vi "Write Mutation Type.vi"(8 "error in (no error)":errorcluster, 10 "Mutation Type":T1, 11 "GA in":refnum<class "GA.lvclass">) -> (0 "error out":errorcluster, 3 "GA out":refnum<class "GA.lvclass">)   [LabVIEW 2013, in "GA.lvclass"]
uses:
  GA.lvclass
  Controls/Mutation Type.ctl
  GA.lvclass/GA.ctl
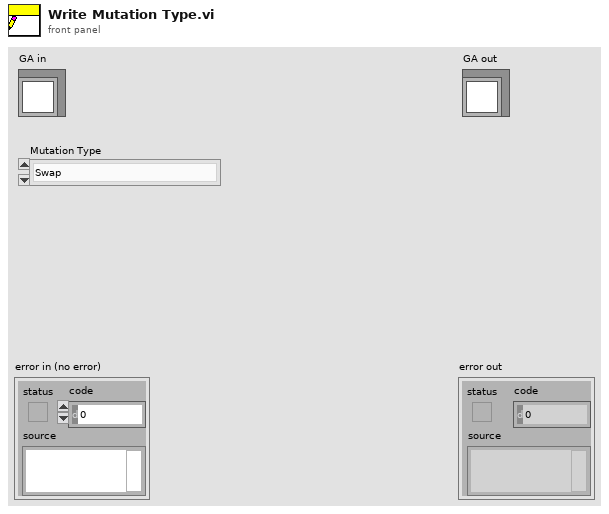
[diagram p1: front panel]
types:
  T1 = typedef "GA.lvclass/Mutation Type.ctl" = enum16{"Swap", "Insert", "Shift", "Shuflle", "Inversion", "ND Mutation"}
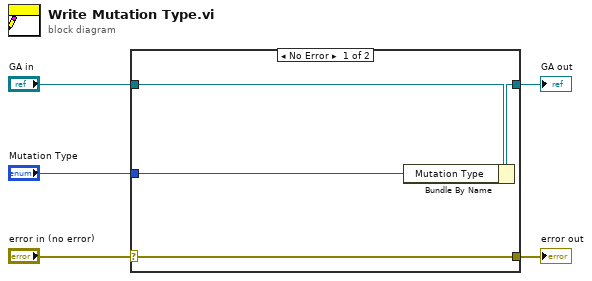
[diagram p0: block diagram]
diagram:
  n1 = case shown="No Error" "error in (no error)" {
    selector: "error in (no error)" -> [w9 w10]
    tunnel: [w9 w10] -> w4
    tunnel: [w7 w11] -> w2
    tunnel: "GA in" -> [w8 w11]
    tunnel: "Mutation Type" -> [w6 _]
    frame No Error {
      n2 = Bundle By Name(cluster=w8, "Mutation Type"=w6) -> (w7:refnum<class "GA.lvclass">)
    }
    frame Error {
    }
  }
  "error out" <- w4
  "GA out" <- w2
